vi "BMM LIN Wait Data Num.vi"(7 "TimeOutMs":i32, 9 "DataNum":u32, 10 "LINIndex":u8, 11 "DevHandle":i32) -> (3 "function return":i32)   [LabVIEW 2010, in "usb2bmm_lin.lvlib"]
doc: "int WINAPI BMM_LIN_WaitDataNum(int DevHandle,unsigned char LINIndex,unsigned int DataNum,int TimeOutMs);"
uses:
  usb2bmm_lin.lvlib
  USB2XXX/trunk/USB2XXX/USB2XXX/vs2019/Release/USB2XXX.dll
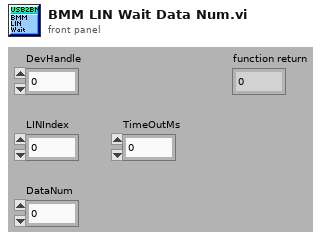
[diagram p1: front panel]
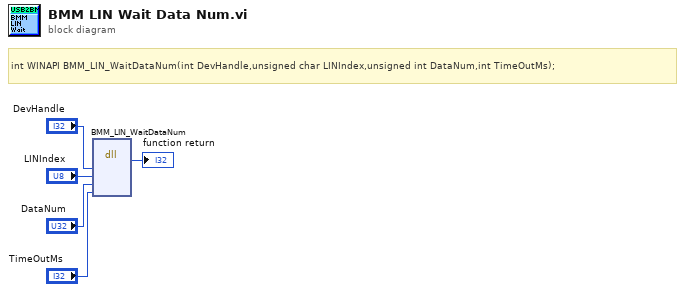
[diagram p0: block diagram]
diagram:
  # "int WINAPI BMM_LIN_WaitDataNum(int DevHandle,unsigned char LINIndex,unsigned int DataNum,int TimeOutMs);"
  n1 = dll-call lib="E:/Projects/USB2XXX/trunk/USB2XXX/USB2XXX/vs2019/Release/USB2XXX.*" fn="BMM_LIN_WaitDataNum"("DevHandle"="DevHandle", "LINIndex"="LINIndex", "DataNum"="DataNum", "TimeOutMs"="TimeOutMs") -> (→"function return":i32)  [unwired: 7 in, 2 out]
